vi "Test Serialize Boolean.vi"(8 "error in (no error)":errorcluster) -> (0 "error out":errorcluster)   [LabVIEW 2013]
uses:
  src/Serializer/JSON Serializer/JSON Serializer.lvclass
  <vilib>/addons/_JKI Toolkits/Caraya/classes/Test/Test.lvclass
  <vilib>/addons/_JKI Toolkits/Caraya/classes/Assert/Assert.lvclass
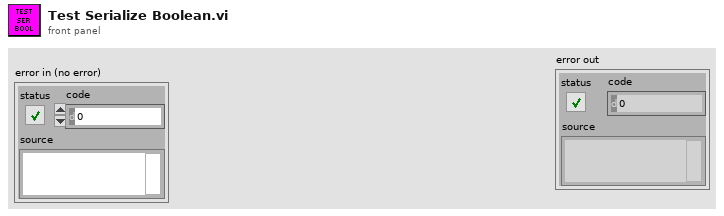
[diagram p1: front panel]
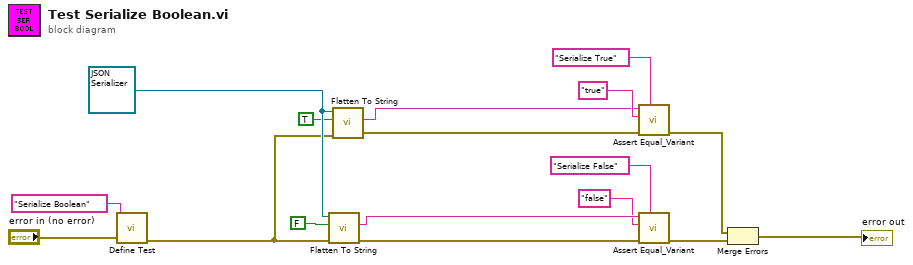
[diagram p0: block diagram]
diagram:
  w7 = refnum<class "JSON Serializer.lvclass"> refnum ("JKI JSON Serialization.lvlib:JSON Serializer.lvclass")
  n1 = call <vilib>:"Define Test.vi"("error in (no error)"="error in (no error)", "Label (VI Title)"="Serialize Boolean") -> ("error out"=w5:errorcluster)  [unwired: 9 in]
  n2 = call-dynamic "Flatten To String.vi"("error in (no error)"=w5, "Variant"=FALSE, "JSON Serializer in"=w7) -> ("error out"=w15:errorcluster, "String"=w13:string)  [unwired: 6 in, 1 out]
  n3 = call-dynamic "Flatten To String.vi"("error in (no error)"=w5, "Variant"=TRUE, "JSON Serializer in"=w7) -> ("error out"=w4:errorcluster, "String"=w3:string)  [unwired: 6 in, 1 out]
  n4 = call <vilib>:"Assert Equal_Variant.vi"("Label"="Serialize True", "error in (no error)"=w4, "Y"="true", "X"=w3) -> ("error out"=w1:errorcluster)  [unwired: 7 in]
  n5 = call <vilib>:"Assert Equal_Variant.vi"("Label"="Serialize False", "error in (no error)"=w15, "Y"="false", "X"=w13) -> ("error out"=w14:errorcluster)  [unwired: 7 in]
  n6 = Merge Errors(w1, w14) -> (→"error out":errorcluster)
